vi "Align and Compress TitleBar Buttons.vi"(8 "Error In":errorcluster, 10 "Button Full Names":string[](array[string]), 11 "Appearance Actor in":refnum<class "Appearance Actor.lvclass">) -> (0 "Error Out":errorcluster, 3 "Appearance Actor out":refnum<class "Appearance Actor.lvclass">)   [LabVIEW 2021, in "Appearance Actor.lvlib" / "Appearance Actor.lvclass"]
uses:
  Appearance Actor.lvclass
  Appearance Actor.lvclass/Appearance Actor.ctl
  <vilib>/regexp/Match Regular Expression.xnode
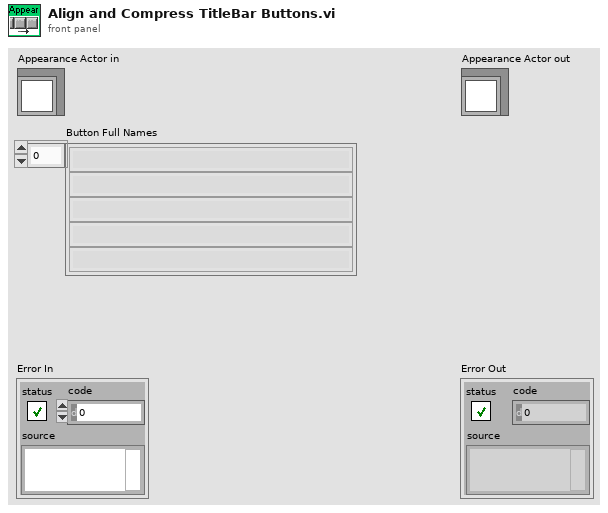
[diagram p1: front panel]
types:
  T1 = typedef "Appearance Actor.lvlib/Appearance Actor.lvclass/UI Controls--map.ctl" = map{string, T2}
  T2 = typedef "Appearance Actor.lvlib/Appearance Actor.lvclass/Element Controls--map.ctl" = map{string, T3}
  T3 = typedef "Appearance Actor.lvlib/Appearance Actor.lvclass/Controls--map.ctl" = map{string, refnum<vi>}
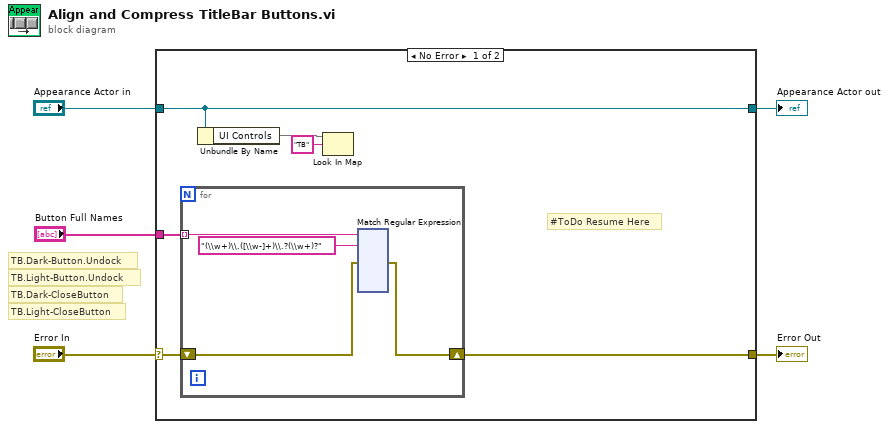
[diagram p0: block diagram]
diagram:
  # "TB.Light-CloseButton"
  # "TB.Dark-CloseButton"
  # "TB.Light-Button.Undock"
  # "TB.Dark-Button.Undock"
  n1 = case shown="No Error" "Error In" {
    selector: "Error In" -> [w8 w138]
    tunnel: [w7 w138] -> w4
    tunnel: [w11 w137] -> w2
    tunnel: "Appearance Actor in" -> [w11 w137]
    tunnel: "Button Full Names" -> [w6 _]
    frame No Error {
      # "#ToDo Resume Here"
      n2 = for {
        tunnel: w6 -> [w12] mode=indexing
        shift-right: [w13] -> w7
        shift-left: w8 -> [w14]
        n3 = xnode "Match Regular Expression"("input string"=w12, "regular expression"="(\\w+)\\.([\\w-]+)\\.?(\\w+)?", "error in"=w14) -> ("error out"=w13:errorcluster)  [unwired: 3 in, 7 out]
      }
      n4 = Unbundle By Name(w11) -> ("UI Controls"=w10:T1)
      n5 = Look In Map(map=w10, key="TB") -> ()  [unwired: 1 in, 2 out]
    }
    frame Error {
    }
  }
  "Error Out" <- w4
  "Appearance Actor out" <- w2
